vi "ADC_Trigger.vi"(8 "error in (no error)":errorcluster, 9 "level %(1.00)":sgl=1.0 min=-100 max=100 step=1, 10 "trigger slope":enum16{"Rising", "Falling"}(ring), 11 "Trigger Source":T1(ring)) -> (0 "error out":errorcluster, 1 "level%":i32, 2 "Level string":string, 3 "Trigger string":string)   [LabVIEW 2010]
doc: "This VI configures the trigger conditions for starting the scan."
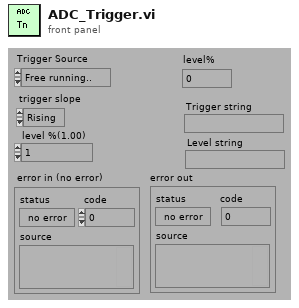
[diagram p1: front panel]
types:
  T1 = enum16{"Free running..", "GPIB GET", "External TTL", "First Channel", "One shot on TALK", "On shot on GET", "One shot TTL"}
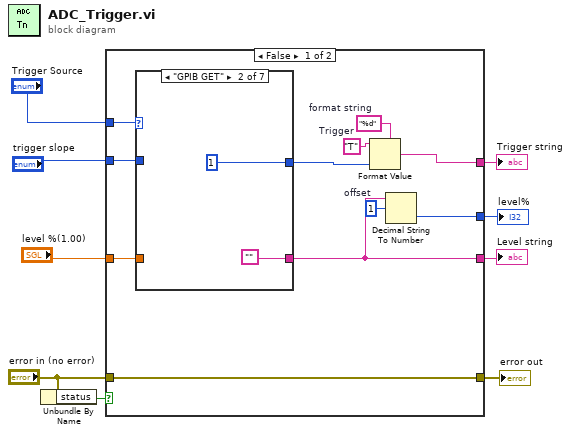
[diagram p0: block diagram]
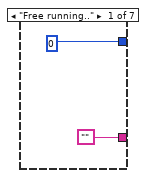
[diagram p2: hidden frame]
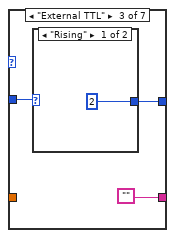
[diagram p3: hidden frame]
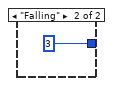
[diagram p4: hidden frame]
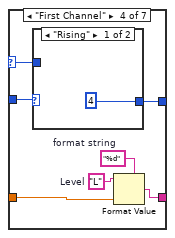
[diagram p5: hidden frame]
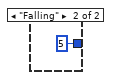
[diagram p6: hidden frame]
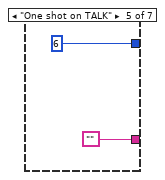
[diagram p7: hidden frame]
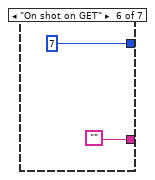
[diagram p8: hidden frame]
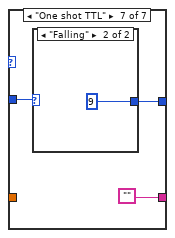
[diagram p9: hidden frame]
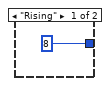
[diagram p10: hidden frame]
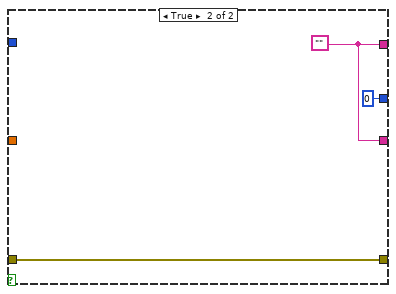
[diagram p11: hidden frame]
diagram:
  n1 = Unbundle By Name("error in (no error)") -> ("status"=w7:bool)
  n2 = case shown="False" w7 {
    tunnel: [w10 w50] -> w9
    tunnel: "error in (no error)" -> [w10 w50]
    tunnel: "Trigger Source" -> [w19 _]
    tunnel: "trigger slope" -> [w18 _]
    tunnel: [w15 w49] -> w4
    tunnel: [w14 w49] -> w3
    tunnel: [w13 0] -> w2
    tunnel: "level %(1.00)" -> [w11 _]
    frame False {
      w12 = 1  # offset
      w16 = "T"  # Trigger
      w20 = "%d"  # format string
      n3 = case shown="\"GPIB GET\"" w19 {
        selector: w19 -> [_ _ _ w35 _ _ _]
        tunnel: w18 -> [_ _ w27 w36 _ _ w45]
        tunnel: [0 1 w26 w34 6 7 w44] -> w17
        tunnel: ["" "" "" w31 "" "" ""] -> w14
        tunnel: w11 -> [_ _ _ w30 _ _ _]
        frame "Free running.." {
        }
        frame "GPIB GET" {
        }
        frame "External TTL" {
          n4 = case shown="\"Rising\"" w27 {
            tunnel: [2 3] -> w26
            frame "Rising" {
            }
            frame "Falling" {
            }
          }
        }
        frame "First Channel" {
          w32 = "%d"  # format string
          w33 = "L"  # Level
          n5 = case shown="\"Rising\"" w36 {
            tunnel: w35 -> [_ _]
            tunnel: [4 5] -> w34
            frame "Rising" {
            }
            frame "Falling" {
            }
          }
          n6 = Format Value(string ("")=w33, format string=w32, value (0)=w30) -> (output string=w31:string)
        }
        frame "One shot on TALK" {
        }
        frame "On shot on GET" {
        }
        frame "One shot TTL" {
          n7 = case shown="\"Falling\"" w45 {
            tunnel: [8 9] -> w44
            frame "Rising" {
            }
            frame "Falling" {
            }
          }
        }
      }
      n8 = Format Value(string ("")=w16, format string=w20, value (0)=w17) -> (output string=w15:string)
      n9 = Decimal String To Number(string=w14, offset=w12) -> (number=w13:i32)  [unwired: 2 out]
    }
    frame True {
      w49 = ""
    }
  }
  "error out" <- w9
  "level%" <- w2
  "Level string" <- w3
  "Trigger string" <- w4
